vi "变形.vi"(11 "数值":i8) -> (3 "数值 2":i8)   [LabVIEW 2012]
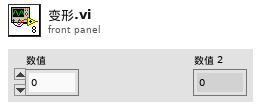
[diagram p1: front panel]
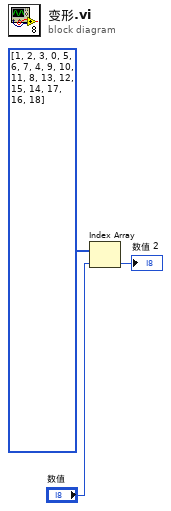
[diagram p0: block diagram]
diagram:
  n1 = Index Array(array=i32[] [1, 2, 3, 0, 5, 6, 7, 4, 9, 10, 11, 8, 13, 12, 15, 14, 17, 16, 18], index="数值") -> (element=→"数值 2":i32)
